vi "Insert Command Event.vi"(8 "error in (no error)":errorcluster, 10 "CmdEvent":refnum<user-event>, 11 "GUI Facade in":refnum<class "GUI Facade.lvclass">) -> (0 "error out":errorcluster, 3 "GUI Facade out":refnum<class "GUI Facade.lvclass">)   [LabVIEW 2015, in "GUI Facade.lvclass"]
uses:
  GUI Facade.lvclass
  Commands/Command.lvclass
  GUI Facade.lvclass/GUI Facade.ctl
  GUI.lvclass/GUI.ctl
  GUI.lvclass
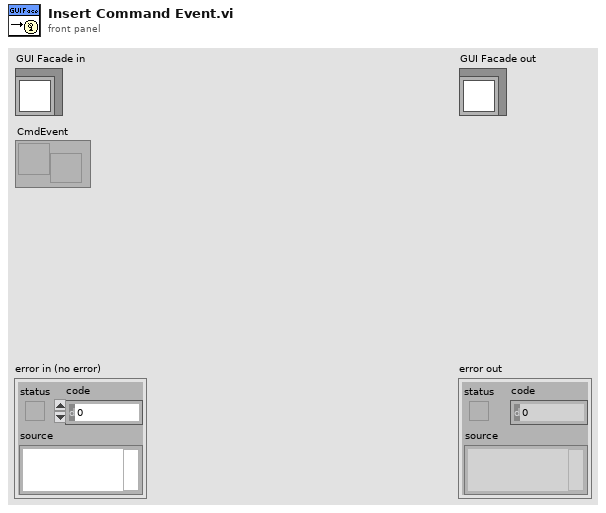
[diagram p1: front panel]
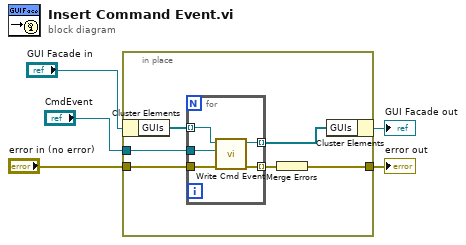
[diagram p0: block diagram]
diagram:
  n1 = in-place {
    in-place-border: "CmdEvent" -> [w10]
    in-place-border: "error in (no error)" -> [w8]
    in-place-border: [w6] -> w1
    n2 = in-place-cluster #1("GUI Facade in") -> ("GUIs"=w11:refnum<class "GUI.lvclass">[])
    n3 = for {
      tunnel: w11 -> [w16] mode=indexing
      tunnel: w10 -> [w15]
      tunnel: [w14] -> w9 mode=indexing
      tunnel: w8 -> [w13]
      tunnel: [w12] -> w7 mode=indexing
      n4 = call "Write Cmd Event.vi"("error in (no error)"=w13, "Cmd Event"=w15, "GUI in"=w16) -> ("error out"=w12:errorcluster, "GUI out"=w14:refnum<class "GUI.lvclass">)  [unwired: 7 in]
    }
    n5 = Merge Errors(w7) -> (w6:errorcluster)
    n6 = in-place-cluster #1("GUIs"=w9) -> (→"GUI Facade out":refnum<class "GUI Facade.lvclass">)
  }
  "error out" <- w1
